vi "LoadProject.vi"(8 "error in (no error)":errorcluster, 10 "Project File Path":path, 11 "ProjectController in":refnum<class "ProjectController.lvclass">) -> (0 "error out":errorcluster, 3 "ProjectController out":refnum<class "ProjectController.lvclass">)   [LabVIEW 2015, in "ProjectController.lvclass"]
uses:
  ProjectController.lvclass
  ProjectController.lvclass/ProjectController.ctl
  Brower Console/Models/BrowerFactory/Interface/Factory.lvclass
  Brower Console/Controllers/Messages/Import BrowerComponent_Msg/Import BrowerComponent_Msg.lvclass/Import BrowerComponent_Msg.ctl
  <vilib>/ActorFramework/Message Enqueuer/Message Enqueuer.lvclass/Message Enqueuer.ctl
  <vilib>/ActorFramework/Message Enqueuer/Enqueue.vi
  <vilib>/ActorFramework/Message Priority Queue/Priority Enqueue.vi
  Brower Console/Controllers/Messages/Import BrowerComponent_Msg/Import BrowerComponent_Msg.lvclass
  Brower Console/Models/BrowerComponent/BrowerComponent/BrowerComponent.lvclass
  Brower Console/Models/Iterator/Interface/Iterator.lvclass
  Models/ProjectManager/XML Project.lvclass
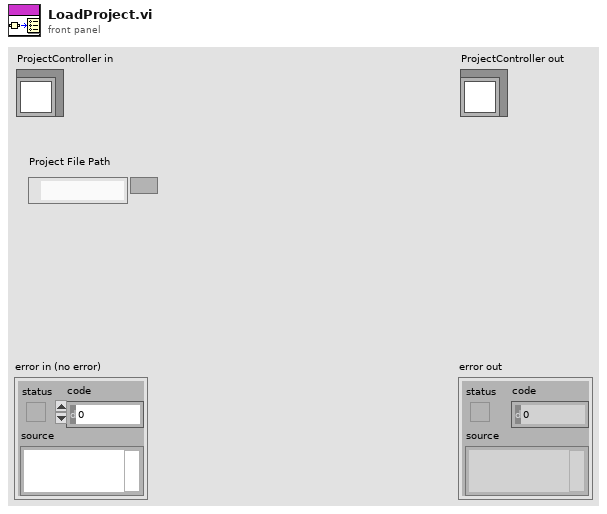
[diagram p1: front panel]
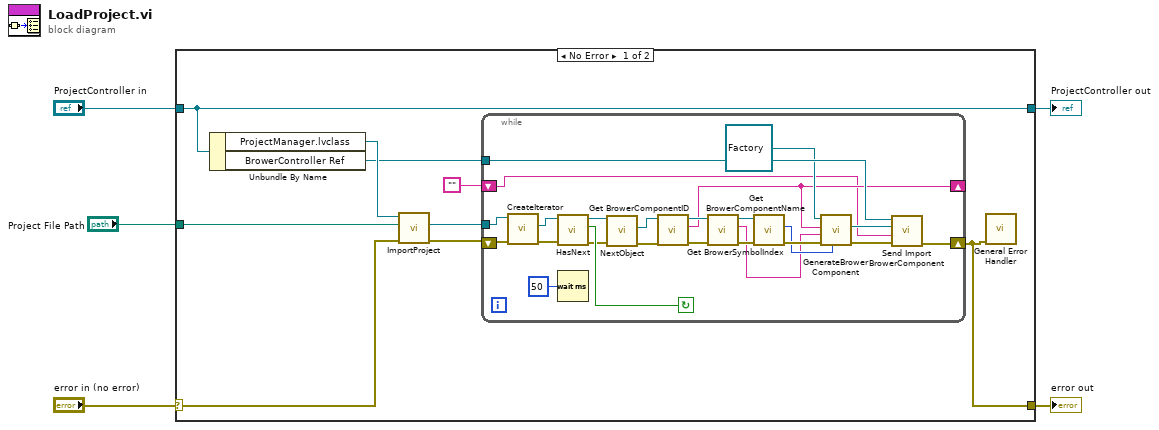
[diagram p0: block diagram]
diagram:
  n1 = case shown="No Error" "error in (no error)" {
    selector: "error in (no error)" -> [w11 w40]
    tunnel: [w6 w40] -> w4
    tunnel: [w14 w39] -> w2
    tunnel: "ProjectController in" -> [w14 w39]
    tunnel: "Project File Path" -> [w12 _]
    frame No Error {
      n2 = Unbundle By Name(w14) -> ("ProjectManager.lvclass"=w13:refnum<class "XML Project.lvclass">, "BrowerController Ref"=w8:refnum<class "Message Enqueuer.lvclass">)
      n3 = call "ImportProject.vi"("error in (no error)"=w11, "XML File Path"=w12, "ProjectManager in"=w13) -> ("error out"=w9:errorcluster, "value"=w10:refnum<class "BrowerComponent.lvclass">)  [unwired: 6 in, 1 out]
      n4 = while {
        tunnel: w10 -> [w37]
        tunnel: w8 -> [w22]
        shift-right: [w18] -> _
        shift-left: "" -> [w17]
        shift-right: [w15] -> w6
        shift-left: w9 -> [w38]
        stop <- w34 continue-if-true
        n5 = call-dynamic "CreateIterator.vi"("error in (no error)"=w38, "BrowerComponent in"=w37) -> ("error out"=w35:errorcluster, "Iterator"=w36:refnum<class "Iterator.lvclass">)  [unwired: 7 in, 1 out]
        n6 = call-dynamic "HasNext.vi"("error in (no error)"=w35, "Iterator"=w36) -> ("error out"=w32:errorcluster, "HasNext?(False)"=w34:bool, "Iterator out"=w33:refnum<class "Iterator.lvclass">)  [unwired: 7 in]
        n7 = Wait (ms)(milliseconds to wait=u32 50) -> ()  [unwired: 1 out]
        n8 = call-dynamic "NextObject.vi"("error in (no error)"=w32, "Iterator"=w33) -> ("error out"=w30:errorcluster, "BrowerComponent"=w31:refnum<class "BrowerComponent.lvclass">)  [unwired: 7 in, 1 out]
        n9 = call "Get BrowerComponentID.vi"("error in (no error)"=w30, "BrowerComponent in"=w31) -> ("error out"=w28:errorcluster, "ComponentID"=w18:string, "BrowerComponent out"=w29:refnum<class "BrowerComponent.lvclass">)  [unwired: 7 in]
        n10 = call "Get BrowerComponentName.vi"("error in (no error)"=w28, "BrowerComponent in"=w29) -> ("error out"=w26:errorcluster, "ComponentName"=w19:string, "BrowerComponent out"=w27:refnum<class "BrowerComponent.lvclass">)  [unwired: 7 in]
        n11 = call "Get BrowerSymbolIndex.vi"("error in (no error)"=w26, "BrowerComponent in"=w27) -> ("error out"=w24:errorcluster, "SymbolIndex"=w23:i32)  [unwired: 7 in, 1 out]
        n12 = call "GenerateBrowerComponent.vi"("SymbolIndex(0)"=w23, "error in (no error)"=w24, "ComponentName(\"\")"=w19, "ComponentID(\"\")"=w18, "Factory in"=refnum<class "Factory.lvclass"> refnum) -> ("error out"=w16:errorcluster, "BrowerComponent"=w21:refnum<class "BrowerComponent.lvclass">)  [unwired: 4 in, 1 out]
        n13 = call "Send Import BrowerComponent.vi"("error in (no error)"=w16, "Parent Tag(\"\")"=w17, "BrowerComponent in"=w21, "Message Enqueuer"=w22) -> ("error out"=w15:errorcluster)  [unwired: 6 in, 1 out]
      }
      n14 = call <vilib>:"General Error Handler.vi"("error in (no error)"=w6) -> ()  [unwired: 10 in, 5 out]
    }
    frame Error {
    }
  }
  "error out" <- w4
  "ProjectController out" <- w2
